vi "Set App.vi"(8 "error in (no error)":errorcluster, 10 "App":refnum<class "ViaApp.lvclass">, 11 "AppDetailPanel in":refnum<class "AppDetailPanel.lvclass">) -> (0 "error out":errorcluster, 3 "AppDetailPanel out":refnum<class "AppDetailPanel.lvclass">)   [LabVIEW 2020, in "PicoG-App.lvlib" / "AppDetailPanel.lvclass"]
uses:
  AppDetailPanel.lvclass
  ViaApp/ViaApp.lvclass
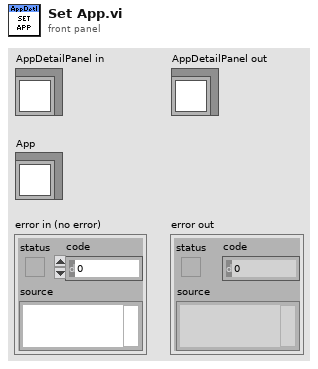
[diagram p1: front panel]
types:
  T1 = typedef "PicoG-App.lvlib/AppDetailPanel.lvclass/Ref Data.ctl" = cluster{"App":refnum<class "ViaApp.lvclass">}
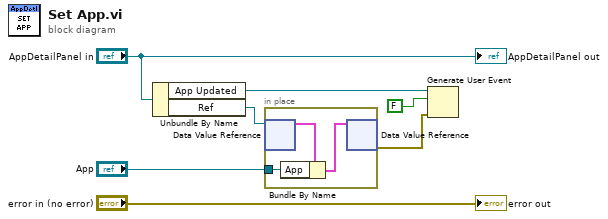
[diagram p0: block diagram]
diagram:
  n1 = Unbundle By Name("AppDetailPanel in") -> ("App Updated"=w3:refnum<user-event>, "Ref"=w6:refnum<data-value>)
  n2 = in-place {
    in-place-border: "App" -> [w8]
    n3 = in-place-dvr #1(w6) -> (w10:T1)  [unwired: 1 out]
    n4 = Bundle By Name(cluster=w10, "App"=w8) -> (w9:T1)
    n5 = in-place-dvr #1(w9) -> (w2:errorcluster)  [unwired: 1 out]
  }
  n6 = Generate User Event(user event=w3, event data cluster=FALSE ("event data"), error in=w2) -> ()  [unwired: 1 in, 2 out]
  "error out" <- "error in (no error)"
  "AppDetailPanel out" <- "AppDetailPanel in"
